vi "turn_offset.vi"(2 "x2":dbl, 3 "x1":dbl, 4 "y2":dbl, 5 "y1":dbl) -> (0 "dis_":dbl, 1 "zeta":dbl)   [LabVIEW 2017]
uses:
  GlobalVar.vi
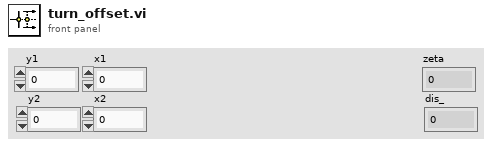
[diagram p1: front panel]
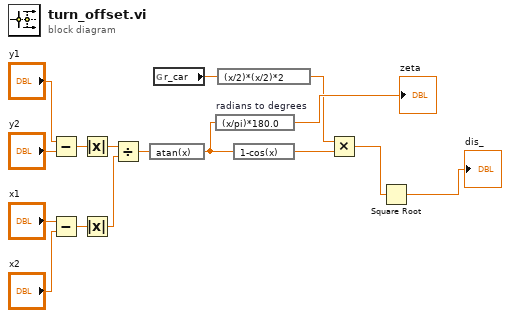
[diagram p0: block diagram]
diagram:
  n1 = Subtract(x="y1", y="y2") -> (x-y=w12:dbl)
  n2 = Subtract(x="x1", y="x2") -> (x-y=w11:dbl)
  n3 = Absolute Value(x=w12) -> (abs(x)=w10:dbl)
  n4 = Absolute Value(x=w11) -> (abs(x)=w9:dbl)
  n5 = Divide(x=w10, y=w9) -> (x/y=w8:dbl)
  n6 = expression code="atan(x)"(w8) -> (w5:dbl)
  n7 = global read "GlobalVar.vi" "r_car"() -> (w6:dbl)
  n8 = expression code="(x/pi)*180.0" "radians to degrees"(w5) -> (→"zeta":dbl)
  n9 = expression code="(x/2)*(x/2)*2"(w6) -> (w3:dbl)
  n10 = expression code="1-cos(x)"(w5) -> (w4:dbl)
  n11 = Multiply(x=w3, y=w4) -> (x*y=w2:dbl)
  n12 = Square Root(x=w2) -> (sqrt(x)=→"dis_":dbl)
